vi "Check if Actuator is Ready.vi"(8 "error in":errorcluster, 10 "Actuator name":string, 11 "UTP IO Session in":T1) -> (0 "error out":errorcluster, 2 "Actuator Ready?":bool, 3 "UTP IO Session out":T1)   [LabVIEW 2023, in "Actuators.lvlib"]
uses:
  Actuators.lvlib
  <vilib>/Noffz/UTP IO/UTP IO Library/Typedefs/Session Handle.ctl
  <vilib>/Noffz/UTP IO/UTP IO Library/UTP IO Pool Session.lvclass
  <vilib>/Noffz/UTP IO/UTP IO Library/methods/poly/plc/Read PLC Variable (Boolean).vi
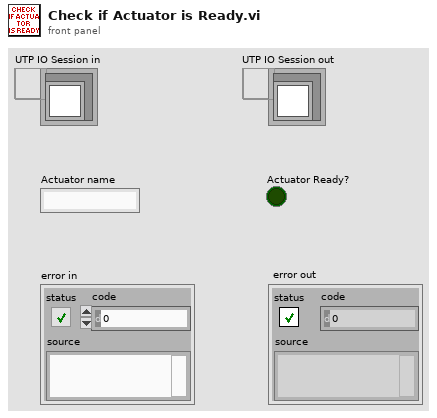
[diagram p1: front panel]
types:
  T1 = typedef "UTP IO Library.lvlib/UTP IO Pool Session.lvclass/Session Handle.ctl" = refnum<data-value>
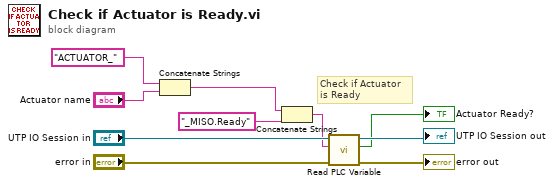
[diagram p0: block diagram]
diagram:
  # "Check if Actuator \nis Ready"
  n1 = Concatenate Strings("ACTUATOR_" ("string"), "Actuator name") -> (w4:string)
  n2 = Concatenate Strings(w4, "_MISO.Ready" ("string")) -> (w6:string)
  n3 = call-poly <vilib>:"Read PLC Variable.vi"("error in (no error)"="error in", "variable name"=w6, "UTP IO Session in"="UTP IO Session in") -> ("error out"=→"error out":errorcluster, "value"=→"Actuator Ready?":bool, "UTP IO Session out"=→"UTP IO Session out":T1)  [unwired: 6 in]
